vi "3D Robot Model.vi"() -> (1 "robot frame":refnum<vi>, 2 "axles":refnum<vi>[](array[refnum]))   [LabVIEW 2017]
uses:
  <vilib>/robotics/Steering/Mecanum Wheel/Roller Orientation.ctl
  <vilib>/robotics/Steering/Utilities/3D Picture/Mecanum Wheel Dimensions.ctl
  <vilib>/robotics/Steering/Utilities/3D Picture/Mecanum Wheel Colors.ctl
  Robot Parameters/Robot Parameters.vi
  <vilib>/picture/3D Picture Control/NI_3D Picture Control.lvlib
  <vilib>/robotics/Steering/Utilities/3D Picture/NI_Robotics 3D Picture Steering Utilities.lvlib
  <vilib>/robotics/Steering/Mecanum Wheel/NI_Robotics_Mecanum Wheel.lvclass
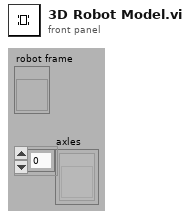
[diagram p1: front panel]
types:
  T1 = typedef "NI_Robotics 3D Picture Steering Utilities.lvlib/Mecanum Wheel Dimensions.ctl" = cluster{"roller thickness":dbl, "roller radius":dbl, "frame thickness":dbl, "number of rollers":i32, "axle radius":dbl, "axle length":dbl}
  T2 = typedef "NI_Robotics_Mecanum Wheel.lvclass/Roller Orientation.ctl" = u16
  T3 = typedef "NI_Robotics 3D Picture Steering Utilities.lvlib/Mecanum Wheel Colors.ctl" = cluster{"wheel color":u32, "roller color":u32}
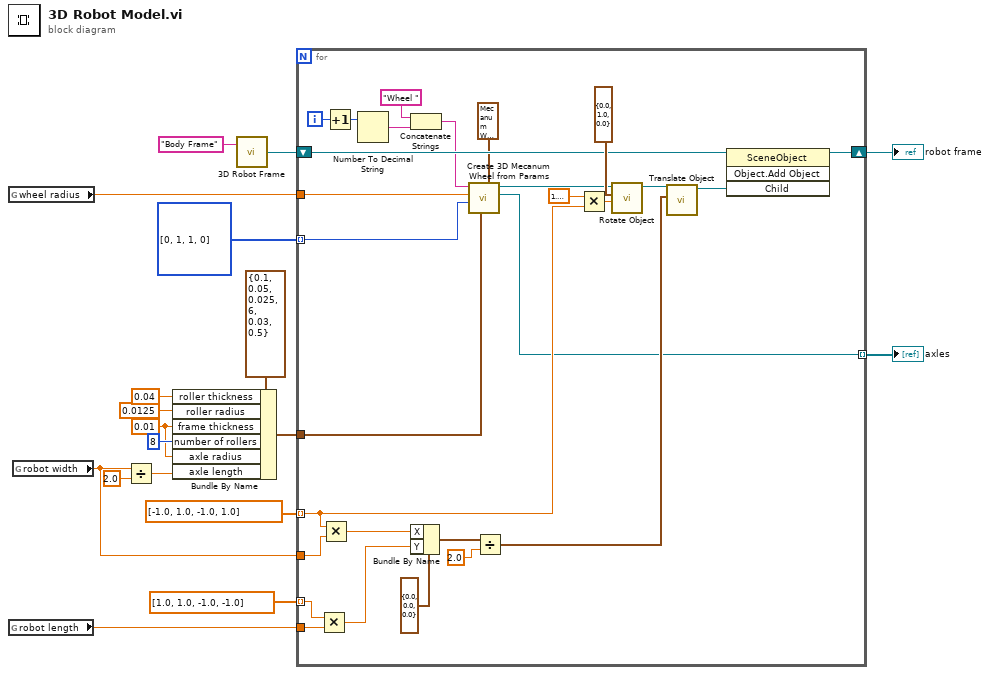
[diagram p0: block diagram]
diagram:
  w6 = 0.01 ("frame thickness")
  w12 = T2[] [0, 1, 1, 0] items=["Left", "Right"]
  n1 = global read "Robot Parameters.vi" "wheel radius"() -> (w3:dbl)
  n2 = global read "Robot Parameters.vi" "robot length"() -> (w1:dbl)
  n3 = global read "Robot Parameters.vi" "robot width"() -> (w2:dbl)
  n4 = Divide(x=w2, y=2.0) -> (x/y=w4:dbl)
  n5 = Bundle By Name(cluster=T1 {"roller thickness"=0.1, "roller radius"=0.05, "frame thickness"=0.025, "number of rollers"=6, "axle radius"=0.03, "axle length"=0.5} ("drawing parameters"), "roller thickness"=0.04, "roller radius"=0.0125, "frame thickness"=w6, "number of rollers"=8, "axle radius"=w6, "axle length"=w4) -> (w11:T1)
  n6 = call "3D Robot Frame.vi"("name"="Body Frame" ("Name")) -> ("robot frame"=w16:refnum<vi>)  [unwired: 1 in]
  n7 = for {
    tunnel: sgl[] [-1.0, 1.0, -1.0, 1.0] -> [w40] mode=indexing
    tunnel: sgl[] [1.0, 1.0, -1.0, -1.0] -> [w37] mode=indexing
    tunnel: w2 -> [w39]
    tunnel: w1 -> [w38]
    shift-right: [w31] -> w18
    shift-left: w16 -> [w29]
    tunnel: w3 -> [w22]
    tunnel: [w23] -> w17 mode=indexing
    tunnel: w12 -> [w21] mode=indexing
    tunnel: w11 -> [w20]
    i -> [w46]
    n8 = Multiply(x=w37, y=w38) -> (x*y=w34:dbl)
    n9 = Multiply(x=w40, y=w39) -> (x*y=w35:dbl)
    n10 = Increment(x=w46) -> (x+1=w45:i32)
    n11 = Number To Decimal String(number=w45) -> (decimal integer string=w26:string)  [unwired: 1 out]
    n12 = Concatenate Strings("Wheel " ("Name"), w26) -> (w25:string)
    n13 = Bundle By Name(cluster=cluster{"X":sgl, "Y":sgl, "Z":sgl} {"X"=0.0, "Y"=0.0, "Z"=0.0} ("Translation"), "X"=w35, "Y"=w34) -> (w33:cluster{"X":sgl, "Y":sgl, "Z":sgl})
    n14 = call <vilib>:"Create 3D Mecanum Wheel from Params.vi"("colors"=T3 {"wheel color"=4884736, "roller color"=1891328}, "dimensions"=w20, "roller orientation"=w21, "wheel radius"=w22, "name"=w25) -> ("rotation axis"=w23:refnum<vi>, "3D mecanum wheel frame"=w24:refnum<vi>)  [unwired: 4 in, 1 out]
    n15 = Divide(x=w33, y=sgl 2.0 ("X")) -> (x/y=w28:cluster{"X":sgl, "Y":sgl, "Z":sgl})
    n16 = Multiply(x=1.5707963267948966, y=w40) -> (x*y=w42:dbl)
    n17 = call <vilib>:"Rotate Object.vi"("Angle"=w42, "Axis"=cluster{"X":sgl, "Y":sgl, "Z":sgl} {"X"=0.0, "Y"=1.0, "Z"=0.0} ("Translation"), "Scene.Object In"=w24) -> ("Scene.Object Out"=w32:refnum<vi>)  [unwired: 1 in, 7 out]
    n18 = call <vilib>:"Translate Object.vi"("Translation"=w28, "Scene.Object In"=w32) -> ("Scene.Object Out"=w30:refnum<vi>)  [unwired: 1 in, 8 out]
    n19 = invoke class="SceneObject" method="Object.Add Object"(reference=w29, "Child"=w30) -> (reference out=w31:refnum<vi>)  [unwired: 2 in, 3 out]
  }
  "robot frame" <- w18
  "axles" <- w17
